vi "Execute.vi"(8 "error in (no error)":errorcluster, 10 "System In":refnum<class "abs_System.lvclass">, 11 "Node in":refnum<class "Test Boolean.lvclass">) -> (0 "error out":errorcluster, 1 "Status":T1, 2 "System Out":refnum<class "abs_System.lvclass">, 3 "Node out":refnum<class "Test Boolean.lvclass">)   [LabVIEW 2021, in "BT.lvlib" / "Test Boolean.lvclass"]
uses:
  Test Boolean.lvclass
  C:/Users/Tim/Documents/GitHub/LV_Behaviour_Tree/Source/abs_Type Leaf/abs_Type Leaf.lvclass
  abs_Node/Status.ctl
  abs_System/abs_System.lvclass
  LV_Abstract/Source/Abs_Types/Boolean/Abs_Boolean.lvclass
  C:/Users/Tim/Documents/GitHub/LV_Abstract/Source/Abs_Types/Type/Abs_Type.lvclass
  abs_Type Leaf/abs_Type Leaf.lvclass/abs_Type Leaf.ctl
  Test Boolean.lvclass/Test Boolean.ctl
  abs_Type Leaf/Properties/Read Value Class.vi
  Properties/Read Succeed State .vi
  abs_Type Leaf/Properties/Write Value Class.vi
  LV_Abstract/Source/Abs_Types/Type/Abs_Type.lvclass
  abs_Type Leaf/abs_Type Leaf.lvclass
  abs_Node/abs_Node.lvclass
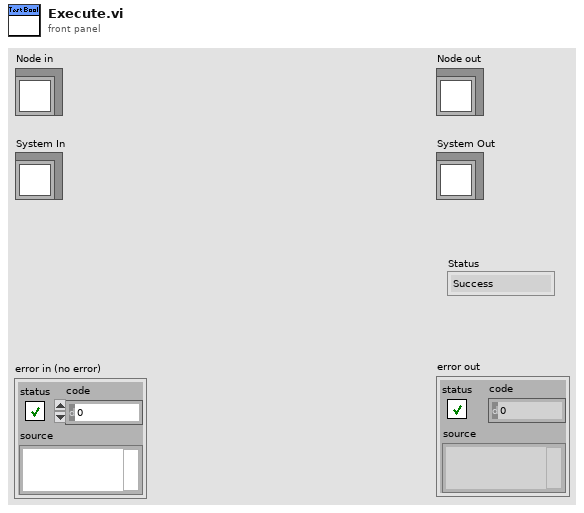
[diagram p1: front panel]
types:
  T1 = typedef "BT.lvlib/abs_Node.lvclass/Status.ctl" = enum16{"Success", "Failure", "Running"}
  T2 = typedef "BT.lvlib/abs_Test Boolean.lvclass/Succeed State.ctl" = enum16{"Succeed on True", "Succeed on Fail"}
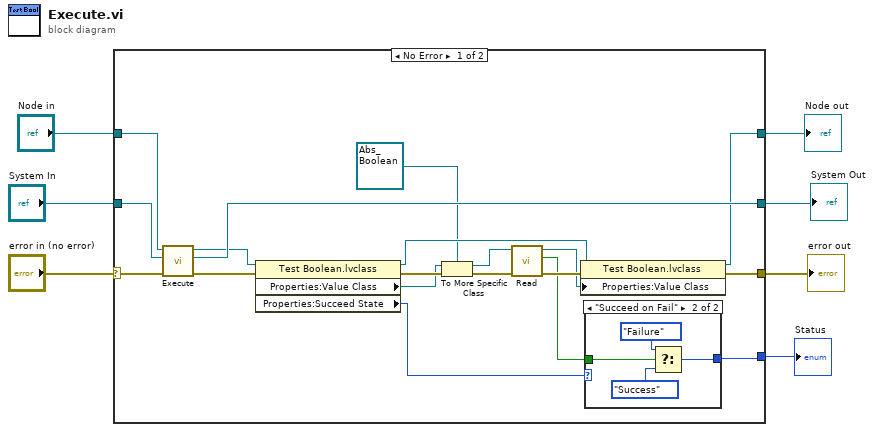
[diagram p0: block diagram]
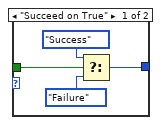
[diagram p2: hidden frame]
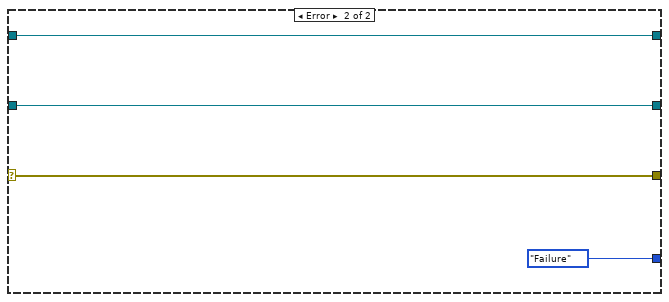
[diagram p3: hidden frame]
diagram:
  n1 = case shown="No Error" "error in (no error)" {
    selector: "error in (no error)" -> [w25 w36]
    tunnel: [w26 w37] -> w3
    tunnel: "System In" -> [w24 w37]
    tunnel: "Node in" -> [w23 w38]
    tunnel: [w19 w36] -> w4
    tunnel: [w18 w38] -> w2
    tunnel: [w16 Status."Failure" ("Status")] -> w1
    frame No Error {
      n2 = call-parent "Execute.vi"("error in (no error)"=w25, "System In"=w24, "Node in"=w23) -> ("error out"=w22:errorcluster, "System Out"=w26:refnum<class "abs_System.lvclass">, "Node out"=w21:refnum<class "Test Boolean.lvclass">)  [unwired: 5 in, 1 out]
      n3 = property class="Test Boolean.lvclass"(reference=w21, error in=w22) -> (reference out=w20:refnum<class "Test Boolean.lvclass">, error out=w12:errorcluster, "Properties:Value Class"=w10:refnum<class "Abs_Type.lvclass">, "Properties:Succeed State "=w17:T2)
      n4 = To More Specific Class(target class=refnum<class "Abs_Boolean.lvclass"> refnum ("Boolean in"), reference=w10, error in=w12) -> (specific class reference=w8:refnum<class "Abs_Boolean.lvclass">, error out=w11:errorcluster)
      n5 = call-dynamic "Read.vi"("error in (no error)"=w11, "Boolean in"=w8) -> ("error out"=w15:errorcluster, "Boolean"=w13:bool, "Boolean out"=w14:refnum<class "Abs_Boolean.lvclass">)  [unwired: 7 in]
      n6 = property class="Test Boolean.lvclass"(reference=w20, error in=w15, "Properties:Value Class"=w14) -> (reference out=w18:refnum<class "Test Boolean.lvclass">, error out=w19:errorcluster)
      n7 = case shown="\"Succeed on Fail\"" w17 {
        tunnel: w13 -> [w29 w33]
        tunnel: [w27 w31] -> w16
        frame "Succeed on True" {
          n8 = Select(t=Status."Success" ("Status"), s=w29, f=Status."Failure" ("Status")) -> (s? t:f=w27:T1)
        }
        frame "Succeed on Fail" {
          n9 = Select(t=Status."Failure" ("Status"), s=w33, f=Status."Success" ("Status")) -> (s? t:f=w31:T1)
        }
      }
    }
    frame Error {
    }
  }
  "error out" <- w4
  "Node out" <- w2
  "Status" <- w1
  "System Out" <- w3
